vi "Set Instrument From Marker.vi"(8 "error in (no error)":errorcluster, 9 "Instrument Setting (0: Reference Level)":u16(ring) items=["Reference Level", "Frequency Center", "Frequency Span", "Frequency Start", "Frequency Stop"], 10 "Marker Number (1)":i32=1, 11 "VISA resource name":refnum<visa-resource-name>) -> (0 "error out":errorcluster, 3 "VISA resource name out":refnum<visa-resource-name>)   [LabVIEW 2013, in "Template - Spectrum Analyzer.lvlib"]
doc: "Sets the reference level or center frequency to the value of the selected marker."
uses:
  <instrlib>/_Template - Spectrum Analyzer/Template - Spectrum Analyzer.lvlib
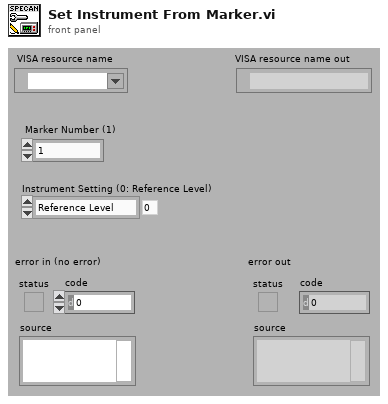
[diagram p1: front panel]
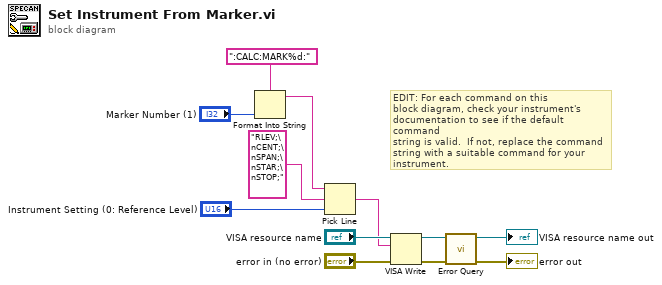
[diagram p0: block diagram]
diagram:
  # "EDIT: For each command on this\nblock diagram, check your instrument's\ndocumentation to see if the default command\nstring is valid.  If not, replace the command\nstring with a suitable command for your\ninstrument."
  n1 = Format Into String(format string=":CALC:MARK%d:" ("initial string"), "Marker Number (1)") -> (resulting string=w6:string)  [unwired: 2 in, 1 out]
  n2 = Pick Line(string ("")=w6, multi-line string="RLEV;\nCENT;\nSPAN;\nSTAR;\nSTOP;", line index="Instrument Setting (0: Reference Level)") -> (output string=w5:string)
  n3 = VISA Write(VISA resource name="VISA resource name", write buffer=w5, error in (no error)="error in (no error)") -> (VISA resource name out=w4:refnum<visa-resource-name>, error out=w2:errorcluster)  [unwired: 1 out]
  n4 = call <instrlib>:"Error Query.vi"("error in (no error)"=w2, "VISA resource name"=w4) -> ("error out"=→"error out":errorcluster, "VISA resource name out"=→"VISA resource name out":refnum<visa-resource-name>)  [unwired: 6 in, 2 out]
